vi "SetColumnPadding.vi"(0 "reference in":refnum<class "DataGridView.lvclass">, 5 "ColumnIndex":i32, 7 "Padding":T1, 11 "error in (no error)":errorcluster) -> (4 "reference out":refnum<class "DataGridView.lvclass">, 15 "error out":errorcluster)   [LabVIEW 2018, in "DataGridView.lvclass"]
doc: "Sets the padding for a specific column index"
uses:
  DataGridView.lvclass
  System.Windows.Forms
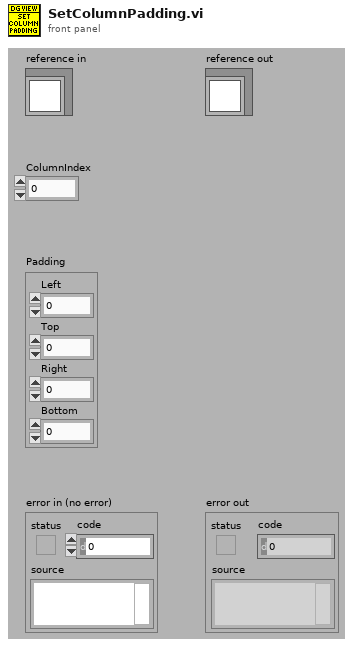
[diagram p1: front panel]
types:
  T1 = cluster{"Left":i32, "Top":i32, "Right":i32, "Bottom":i32}
  T2 = typedef "DataGridView.lvclass/ObjectAttributes.ctl" = cluster{"DataGridView":refnum<k24>, "SelectionChangedEvent":refnum<user-event>, "SelectionChanged callback ref":refnum<k27>, "LastSelectedRowIndex":i32}
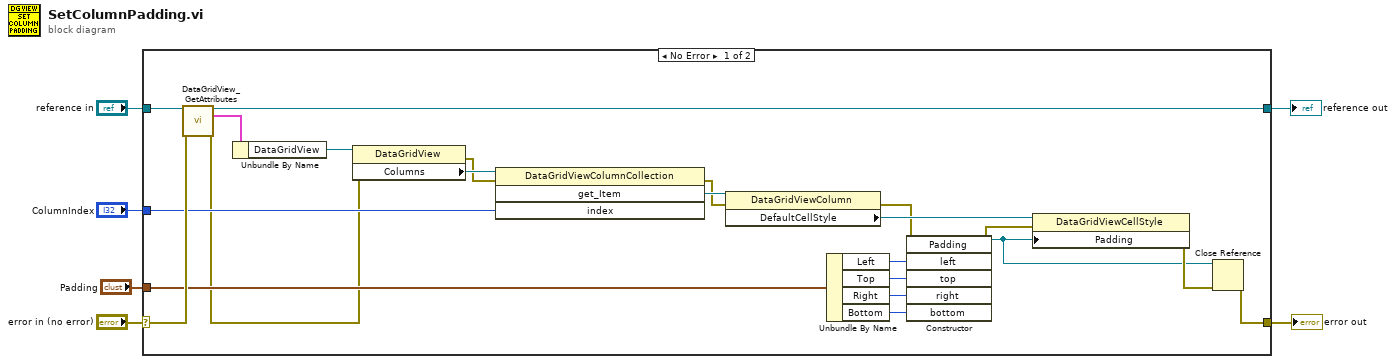
[diagram p0: block diagram]
diagram:
  n1 = case shown="No Error" "error in (no error)" {
    selector: "error in (no error)" -> [w28 w30]
    tunnel: [w8 w30] -> w5
    tunnel: [w25 w29] -> w3
    tunnel: "reference in" -> [w26 w29]
    tunnel: "ColumnIndex" -> [w22 _]
    tunnel: "Padding" -> [w19 _]
    frame No Error {
      n2 = call "DataGridView_GetAttributes.vi"("reference in"=w26, "error in (no error)"=w28) -> ("reference out"=w25:refnum<class "DataGridView.lvclass">, "Data"=w27:T2, "error out"=w9:errorcluster)  [unwired: 10 in, 1 out]
      n3 = Unbundle By Name(w27) -> ("DataGridView"=w24:refnum<k24>)
      n4 = property class="DataGridView"(reference=w24, error in=w9) -> (error out=w14:errorcluster, "Columns"=w23:refnum<k24>)  [unwired: 1 out]
      n5 = invoke class="DataGridViewColumnCollection" method="get_Item"(reference=w23, error in=w14, "index"=w22) -> (error out=w13:errorcluster, "get_Item"=w21:refnum<k24>)  [unwired: 1 in, 2 out]
      n6 = property class="DataGridViewColumn"(reference=w21, error in=w13) -> (error out=w12:errorcluster, "DefaultCellStyle"=w20:refnum<k24>)  [unwired: 1 out]
      n7 = Unbundle By Name(w19) -> ("Left"=w18:i32, "Top"=w17:i32, "Right"=w16:i32, "Bottom"=w15:i32)
      n8 = constructor class="Padding"(error in=w12, "left"=w18, "top"=w17, "right"=w16, "bottom"=w15) -> (reference out=w7:refnum<k24>, error out=w11:errorcluster)  [unwired: 2 in, 5 out]
      n9 = property class="DataGridViewCellStyle"(reference=w20, error in=w11, "Padding"=w7) -> (error out=w10:errorcluster)  [unwired: 1 out]
      n10 = Close Reference(reference=w7, error in (no error)=w10) -> (error out=w8:errorcluster)
    }
    frame Error {
    }
  }
  "error out" <- w5
  "reference out" <- w3
